vi "capex analog out.vi"() -> ()   [LabVIEW 2013]
panel:
  in  "stop":bool
  in  "Update values":bool
  in  "Update labels":bool
  in  "Numeric 16":dbl
  in  "Numeric 15":dbl
  in  "Numeric 14":dbl
  in  "Numeric 13":dbl
  in  "Numeric 12":dbl
  in  "Numeric 11":dbl
  in  "Numeric 10":dbl
  in  "Numeric 9":dbl
  in  "Numeric 8":dbl
  in  "Numeric 7":dbl
  in  "Numeric 6":dbl
  in  "Numeric 5":dbl
  in  "Numeric 4":dbl
  in  "Numeric 3":dbl
  in  "Numeric 2":dbl
  in  "Numeric":dbl
  in  "String 33":string="AO16"
  in  "String 32":string="AO15"
  in  "String 31":string="AO14"
  in  "String 30":string="AO13"
  in  "String 29":string="AO12"
  in  "String 28":string="AO11"
  in  "String 27":string="AO10"
  in  "String 26":string="AO9"
  in  "String 25":string="AO8"
  in  "String 24":string="AO7"
  in  "String 23":string="AO6"
  in  "String 22":string="AO5"
  in  "String 21":string="AO4"
  in  "String 20":string="AO3"
  in  "String 19":string="AO2"
  in  "String 9":string="AO1"
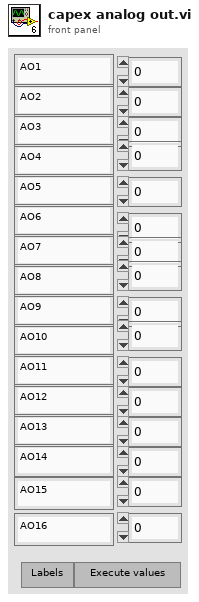
[diagram p1: front panel]
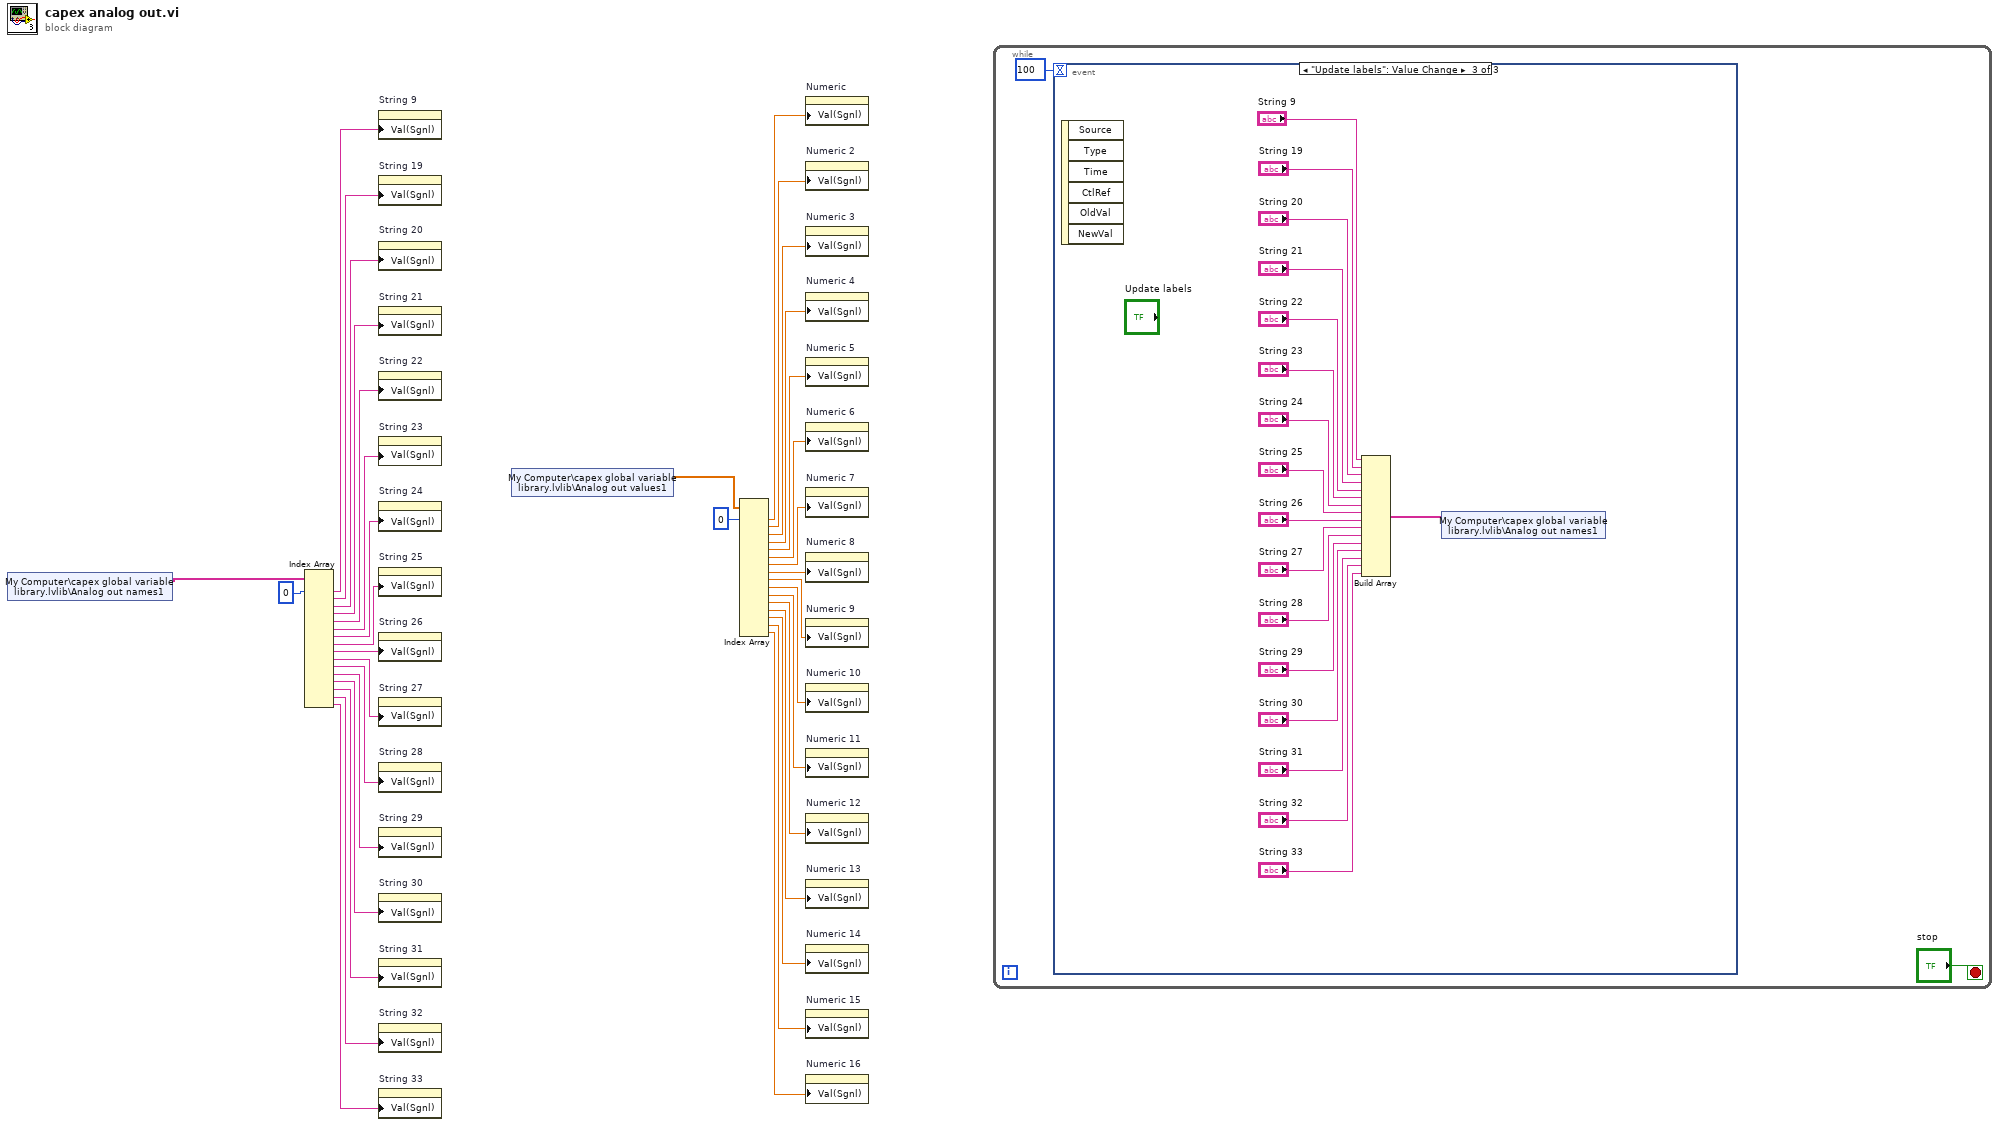
[diagram p0: block diagram]
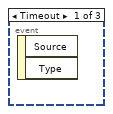
[diagram p2: hidden frame]
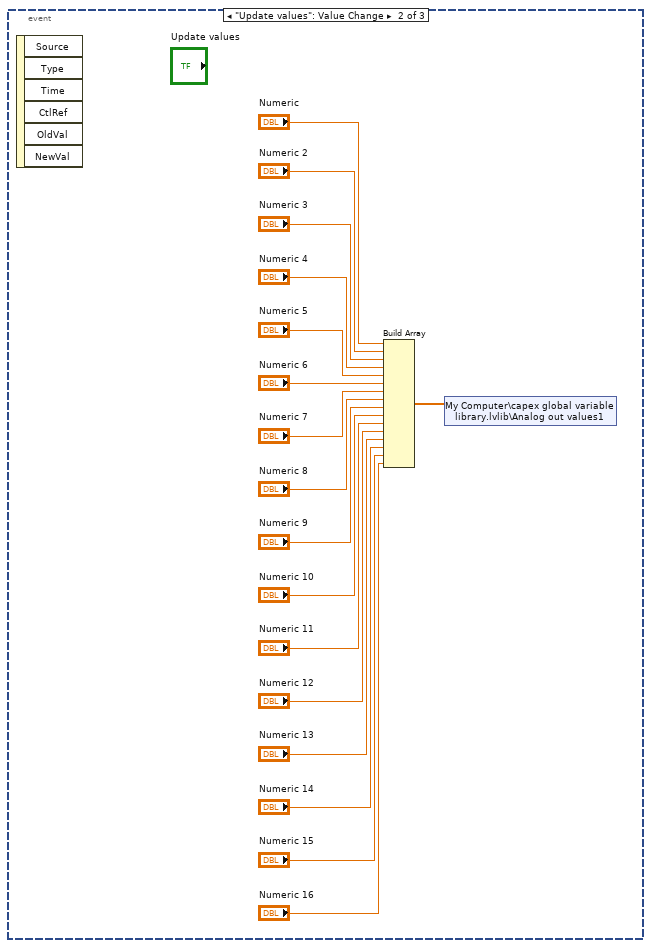
[diagram p3: hidden frame]
diagram:
  n1 = shared-variable "My Computer\\capex global variable library.lvlib\\Analog out names1"() -> (w2:string[])  [unwired: 1 in, 1 out]
  n2 = Index Array(array=w2, index #1=0 ("index")) -> (element #1=w18:string, element #2=w17:string, element #3=w16:string, element #4=w15:string, element #5=w14:string, element #6=w13:string, element #7=w12:string, element #8=w11:string, element #9=w10:string, element #10=w9:string, element #11=w8:string, element #12=w7:string, element #13=w6:string, element #14=w5:string, element #15=w4:string, element #16=w3:string)  [unwired: 15 in]
  n3 = property on="String 9" class="Str"("Val(Sgnl)"=w18) -> ()  [unwired: 2 in, 2 out]
  n4 = property on="String 19" class="Str"("Val(Sgnl)"=w17) -> ()  [unwired: 2 in, 2 out]
  n5 = property on="String 20" class="Str"("Val(Sgnl)"=w16) -> ()  [unwired: 2 in, 2 out]
  n6 = property on="String 21" class="Str"("Val(Sgnl)"=w15) -> ()  [unwired: 2 in, 2 out]
  n7 = property on="String 22" class="Str"("Val(Sgnl)"=w14) -> ()  [unwired: 2 in, 2 out]
  n8 = property on="String 23" class="Str"("Val(Sgnl)"=w13) -> ()  [unwired: 2 in, 2 out]
  n9 = property on="String 24" class="Str"("Val(Sgnl)"=w12) -> ()  [unwired: 2 in, 2 out]
  n10 = property on="String 25" class="Str"("Val(Sgnl)"=w11) -> ()  [unwired: 2 in, 2 out]
  n11 = property on="String 26" class="Str"("Val(Sgnl)"=w10) -> ()  [unwired: 2 in, 2 out]
  n12 = property on="String 27" class="Str"("Val(Sgnl)"=w9) -> ()  [unwired: 2 in, 2 out]
  n13 = property on="String 28" class="Str"("Val(Sgnl)"=w8) -> ()  [unwired: 2 in, 2 out]
  n14 = property on="String 29" class="Str"("Val(Sgnl)"=w7) -> ()  [unwired: 2 in, 2 out]
  n15 = property on="String 30" class="Str"("Val(Sgnl)"=w6) -> ()  [unwired: 2 in, 2 out]
  n16 = property on="String 31" class="Str"("Val(Sgnl)"=w5) -> ()  [unwired: 2 in, 2 out]
  n17 = property on="String 32" class="Str"("Val(Sgnl)"=w4) -> ()  [unwired: 2 in, 2 out]
  n18 = property on="String 33" class="Str"("Val(Sgnl)"=w3) -> ()  [unwired: 2 in, 2 out]
  n19 = shared-variable "My Computer\\capex global variable library.lvlib\\Analog out values1"() -> (w1:dbl[])  [unwired: 1 in, 1 out]
  n20 = Index Array(array=w1, index #1=0 ("index")) -> (element #1=w35:dbl, element #2=w34:dbl, element #3=w33:dbl, element #4=w32:dbl, element #5=w31:dbl, element #6=w30:dbl, element #7=w29:dbl, element #8=w28:dbl, element #9=w27:dbl, element #10=w26:dbl, element #11=w25:dbl, element #12=w24:dbl, element #13=w23:dbl, element #14=w22:dbl, element #15=w21:dbl, element #16=w20:dbl)  [unwired: 15 in]
  n21 = property on="Numeric" class="DigNum (strict)"("Val(Sgnl)"=w35) -> ()  [unwired: 2 in, 2 out]
  n22 = property on="Numeric 2" class="DigNum (strict)"("Val(Sgnl)"=w34) -> ()  [unwired: 2 in, 2 out]
  n23 = property on="Numeric 3" class="DigNum (strict)"("Val(Sgnl)"=w33) -> ()  [unwired: 2 in, 2 out]
  n24 = property on="Numeric 4" class="DigNum (strict)"("Val(Sgnl)"=w32) -> ()  [unwired: 2 in, 2 out]
  n25 = property on="Numeric 5" class="DigNum (strict)"("Val(Sgnl)"=w31) -> ()  [unwired: 2 in, 2 out]
  n26 = property on="Numeric 6" class="DigNum (strict)"("Val(Sgnl)"=w30) -> ()  [unwired: 2 in, 2 out]
  n27 = property on="Numeric 7" class="DigNum (strict)"("Val(Sgnl)"=w29) -> ()  [unwired: 2 in, 2 out]
  n28 = property on="Numeric 8" class="DigNum (strict)"("Val(Sgnl)"=w28) -> ()  [unwired: 2 in, 2 out]
  n29 = property on="Numeric 9" class="DigNum (strict)"("Val(Sgnl)"=w27) -> ()  [unwired: 2 in, 2 out]
  n30 = property on="Numeric 10" class="DigNum (strict)"("Val(Sgnl)"=w26) -> ()  [unwired: 2 in, 2 out]
  n31 = property on="Numeric 11" class="DigNum (strict)"("Val(Sgnl)"=w25) -> ()  [unwired: 2 in, 2 out]
  n32 = property on="Numeric 12" class="DigNum (strict)"("Val(Sgnl)"=w24) -> ()  [unwired: 2 in, 2 out]
  n33 = property on="Numeric 13" class="DigNum (strict)"("Val(Sgnl)"=w23) -> ()  [unwired: 2 in, 2 out]
  n34 = property on="Numeric 14" class="DigNum (strict)"("Val(Sgnl)"=w22) -> ()  [unwired: 2 in, 2 out]
  n35 = property on="Numeric 15" class="DigNum (strict)"("Val(Sgnl)"=w21) -> ()  [unwired: 2 in, 2 out]
  n36 = property on="Numeric 16" class="DigNum (strict)"("Val(Sgnl)"=w20) -> ()  [unwired: 2 in, 2 out]
  n37 = while {
    stop <- "stop" stop-if-true
    n38 = event shown="[2] \"Update labels\": Value Change" {
      selector: _ -> [_ _ _]
      dyn-events: _ -> [_ _ _]
      timeout: 100 -> [_ _ _]
      event Timeout {
        n39 = event-data() -> ()  [unwired: 1 in, 2 out]
      }
      event "Update values": Value Change {
        n40 = event-data() -> ()  [unwired: 1 in, 6 out]
        n41 = Build Array("Numeric", "Numeric 2", "Numeric 3", "Numeric 4", "Numeric 5", "Numeric 6", "Numeric 7", "Numeric 8", "Numeric 9", "Numeric 10", "Numeric 11", "Numeric 12", "Numeric 13", "Numeric 14", "Numeric 15", "Numeric 16") -> (w39:dbl[])
        n42 = shared-variable "My Computer\\capex global variable library.lvlib\\Analog out values1"(w39) -> ()  [unwired: 1 in, 1 out]
      }
      event "Update labels": Value Change {
        n43 = event-data() -> ()  [unwired: 1 in, 6 out]
        n44 = Build Array("String 9", "String 19", "String 20", "String 21", "String 22", "String 23", "String 24", "String 25", "String 26", "String 27", "String 28", "String 29", "String 30", "String 31", "String 32", "String 33") -> (w56:string[])
        n45 = shared-variable "My Computer\\capex global variable library.lvlib\\Analog out names1"(w56) -> ()  [unwired: 1 in, 1 out]
      }
    }
  }
